vi "Erase Firmware.vi"(6 "Remote Timeout (300,000 ms)":u32=300000, 7 "Stop Tasks Automatically (T)":bool=TRUE, 8 "error in (no error)":errorcluster, 11 "Resource in":refnum<k20>) -> (0 "error out":errorcluster, 1 "Firmware Status":T1=2 items=["update pending auto restart"=-4, "verifying new image"=-3, "writing/flashing new image"=-2, "waiting for image"=-1, "corrupt firmware, cannot run"=0, "no firmware installed"=1, "normal operation"=2, "update pending user restart"=3, "update pending user action"=4, "update attempt failed"=5], 2 "Detailed Result":string, 3 "Resource out":refnum<k20>, 4 "Previous Firmware Version":string)   [LabVIEW 2017, in "nisyscfg.lvlib"]
doc: "Removes the firmware image from the resource or target."
uses:
  <vilib>/nisyscfg/nisyscfg.lvlib
  <vilib>/nisyscfg/Firmware Status.ctl
  <vilib>/Utility/error.llb/Error Cluster From Error Code.vi
  <resource>/objmgr/nisysapi.rc
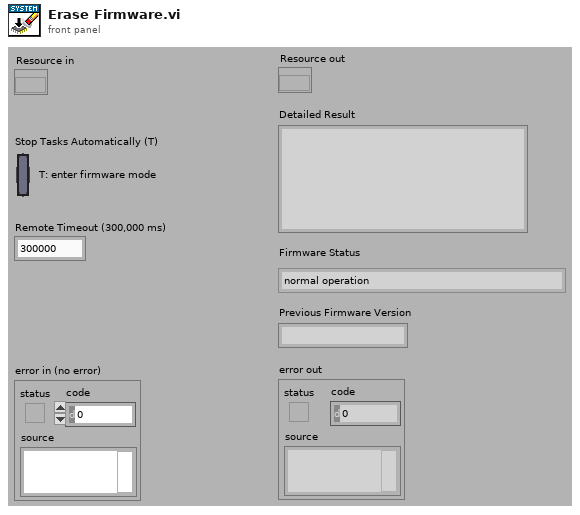
[diagram p1: front panel]
types:
  T1 = typedef "nisyscfg.lvlib/Firmware Status.ctl" = i32
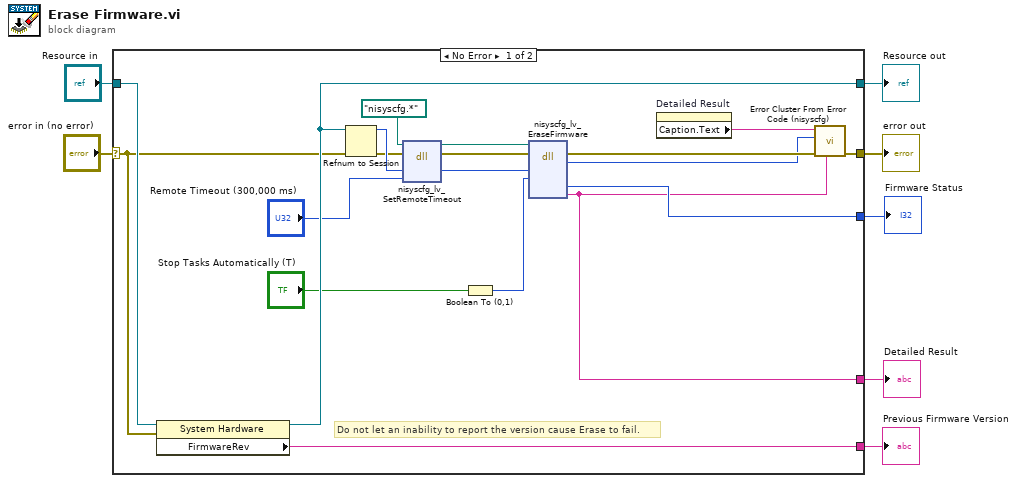
[diagram p0: block diagram]
diagram:
  n1 = case shown="No Error" "error in (no error)" {
    selector: "error in (no error)" -> [w12 w28]
    tunnel: [w11 w28] -> w7
    tunnel: "Resource in" -> [w19 w27]
    tunnel: [w18 w27] -> w4
    tunnel: [w17 _] -> w3
    tunnel: [w13 _] -> w2
    tunnel: [w8 _] -> w1
    frame No Error {
      # "Do not let an inability to report the version cause Erase to fail."
      n2 = property class="System Hardware"(reference=w19, error in=w12) -> (reference out=w18:refnum<k20>, "FirmwareRev"=w17:string)  [unwired: 1 out]
      n3 = Refnum to Session(4:w12, 7:w18) -> (0:w24:errorcluster, 3:w25:u64)
      n4 = dll-call lib="nisyscfg.*" fn="nisyscfg_lv_SetRemoteTimeout" label="SetRemoteTimeout"(path in=path "nisyscfg.*", error in=w24, "item"=w25, "connectTimeout"="Remote Timeout (300,000 ms)") -> (path out=w20:path, error out=w22:errorcluster, "item"=w21:u64)  [unwired: 1 in, 2 out]
      n5 = Boolean To (0,1)(Boolean="Stop Tasks Automatically (T)") -> (0, 1=w14:i16)
      n6 = dll-call lib="nisyscfg.*" fn="nisyscfg_lv_EraseFirmware" label="EraseFirmware"(path in=w20, error in=w22, "itemHandle"=w21, "stopTasks"=w14) -> (error out=w26:errorcluster, "return type"=w9:i32, "firmwareStatus"=w13:i32, "details"=w8:string)  [unwired: 5 in, 1 out]
      n7 = property on="Detailed Result" class="Str"() -> ("Caption.Text"=w10:string)  [unwired: 2 in, 2 out]
      n8 = call <vilib>:"Error Cluster From Error Code (nisyscfg).vi"("Details String"=w8, "error in (no error)"=w26, "Error Code (0)"=w9, "Details Caption"=w10) -> ("error out"=w11:errorcluster)  [unwired: 7 in]
    }
    frame Error {
    }
  }
  "error out" <- w7
  "Resource out" <- w4
  "Previous Firmware Version" <- w3
  "Firmware Status" <- w2
  "Detailed Result" <- w1
